vi "GLdrv_Write_USB.vi"(0 "hDevice":i32, 5 "lpBuffer":string, 11 "error in (no error)":errorcluster, 12 "dwTimeOut":u32) -> (4 "dup hDevice":i32, 8 "lpNumberOfBytesRead":u32, 15 "error out":errorcluster)   [LabVIEW 2017]
uses:
  gtcusbr.dll
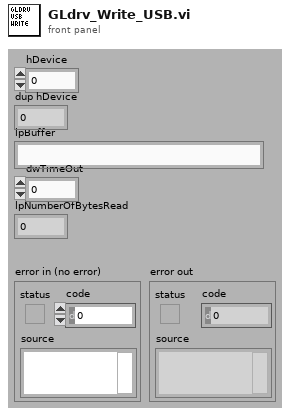
[diagram p1: front panel]
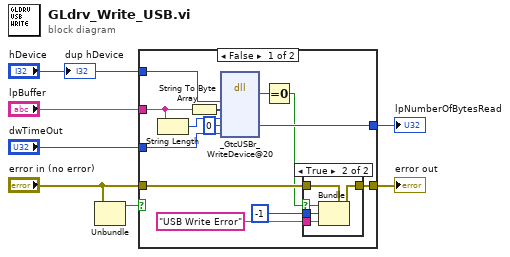
[diagram p0: block diagram]
diagram:
  n1 = Unbundle("error in (no error)") -> ("status"=w1:bool)  [unwired: 2 out]
  n2 = case shown="FALSE" w1 {
    tunnel: "hDevice" -> [w20 _]
    tunnel: [w17 _] -> w6
    tunnel: "dwTimeOut" -> [w16 _]
    tunnel: "lpBuffer" -> [w14 _]
    tunnel: "error in (no error)" -> [w11 w27]
    tunnel: [w12 w27] -> w3
    frame False {
      n3 = String Length(string=w14) -> (length=w15:i32)
      n4 = String To Byte Array(string=w14) -> (unsigned byte array=w13:u8[])
      n5 = dll-call lib="D:/src/LabVIEW/GL860/JP/LabView VI/Driver/gtcusbr.dll" fn="_GtcUSBr_WriteDevice@20"("hDevice"=w20, "lpBuffer"=w13, "nNumberOfBytesToRead"=w15, "lpNumberOfBytesRead"=u32 0, "dwTimeOut"=w16) -> ("BOOL"=w19:i8, "lpNumberOfBytesRead"=w17:u32)  [unwired: 7 in, 2 out]
      n6 = Equal To 0?(x=w19) -> (x = 0?=w8:bool)
      n7 = case shown="TRUE" w8 {
        selector: w8 -> [_ w22]
        tunnel: [w21 w26] -> w12
        tunnel: w11 -> [w21 w25]
        tunnel: "USB Write Error" ("source") -> [_ w24]
        tunnel: -1 ("code") -> [_ w23]
        frame False {
        }
        frame True {
          n8 = Bundle(cluster=w25, "status"=w22, "code"=w23, "source"=w24) -> (w26:errorcluster)
        }
      }
    }
    frame True {
    }
  }
  "lpNumberOfBytesRead" <- w6
  "error out" <- w3
  "dup hDevice" <- "hDevice"
